vi "json_escape.vi"(10 "string":string) -> (2 "escaped string":string)   [LabVIEW 2013, in "Caraya.lvlib" / "MsgSerializer.JSON.lvclass"]
uses:
  MsgSerializer.JSON.lvclass
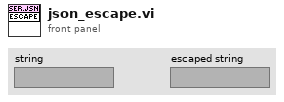
[diagram p1: front panel]
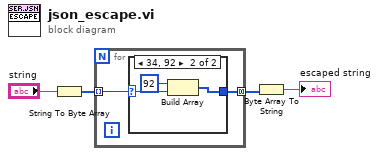
[diagram p0: block diagram]
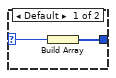
[diagram p2: hidden frame]
diagram:
  n1 = String To Byte Array(string="string") -> (unsigned byte array=w4:u8[])
  n2 = for {
    tunnel: w4 -> [w6] mode=indexing
    tunnel: [w5] -> w3 mode=concatenating
    n3 = case shown="34, 92" w6 {
      selector: w6 -> [w8 w11]
      tunnel: [w7 w10] -> w5
      frame Default {
        n4 = Build Array(w8) -> (w7:u8[])
      }
      frame 34, 92 {
        n5 = Build Array(u8 92 ("element"), w11) -> (w10:u8[])
      }
    }
  }
  n6 = Byte Array To String(unsigned byte array=w3) -> (string=→"escaped string":string)
